vi "poly_run_vi_ref.vi"(8 "Error in":errorcluster caption="Error in (no error)", 9 "Auto dispose VI refnum?":bool=TRUE caption="Auto dispose VI refnum? (T)", 10 "Wait until VI done?":bool caption="Wait until VI done? (F)", 11 "VI refnum in":refnum<vi>) -> (0 "Error out":errorcluster, 1 "Was running?":bool, 2 "VI running?":bool, 3 "VI refnum out":refnum<vi>, 4 "Last execution state":T1(ring))   [LabVIEW 2015, in "_ref_tools_polys.lvlib"]
doc: "Runs the VI that <B>VI refnum in</B> refers to.\n\nThis function will wait until the VI is done if <B>Wait until VI done?</B> is True (default is False), and it will auto dispose the VI reference (hand it over to the running VI) if <B>Auto dispose VI refnum?</B> is True.\n\nThe VI must already be in memory (execution state \"Idle\" or \"Running\") for this function to take any action.\n\nThe <B>VI running?</B> output will only be True if the VI's <B>Last execution state</B> is \"Run top level\". Note that if this function fails to run the VI, <B>VI refnum in</B> will not be auto-disposed, in which case you retain the responsibility of closing that reference yourself.\n\nThis VI is reentrant, and it doesn't run if there is an error on <B>Error in</B>.\n\nSteen Schmidt\nGPower\n30/12 2012"
uses:
  _ref_tools_polys.lvlib
  poly_is_running_state.vi
panel:
  # "Based on Steen Schmidt's GPower"
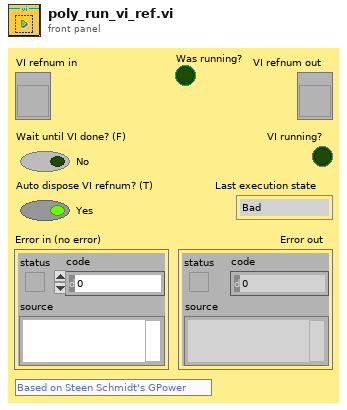
[diagram p1: front panel]
types:
  T1 = enum32{"Bad", "Idle", "Run top level", "Running"}
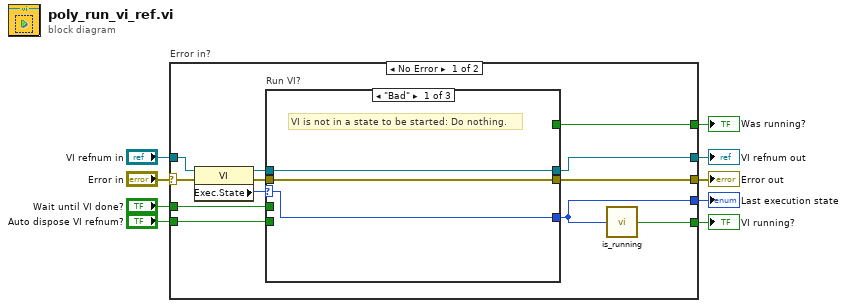
[diagram p0: block diagram]
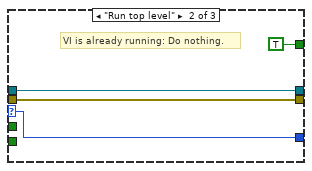
[diagram p2: hidden frame]
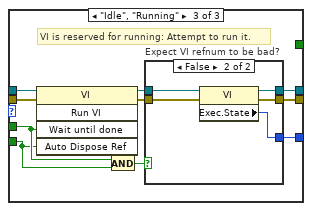
[diagram p3: hidden frame]
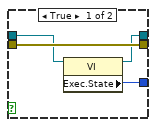
[diagram p4: hidden frame]
diagram:
  n1 = case "Error in?" shown="No Error" "Error in" {
    selector: "Error in" -> [w19 w48]
    tunnel: [w21 w48] -> w8
    tunnel: "VI refnum in" -> [w17 w49]
    tunnel: [w20 w49] -> w6
    tunnel: [w11 _] -> w5
    tunnel: [w10 _] -> w4
    tunnel: "Auto dispose VI refnum?" -> [w14 _]
    tunnel: "Wait until VI done?" -> [w13 _]
    tunnel: [w12 _] -> w1
    frame No Error {
      n2 = property class="VI"(reference=w17, error in=w19) -> (reference out=w16:refnum<vi>, error out=w18:errorcluster, "Exec.State"=w15:T1)
      n3 = case "Run VI?" shown="\"Bad\"" w15 {
        selector: w15 -> [w22 w26 _]
        tunnel: [w24 w28 w35] -> w21
        tunnel: w18 -> [w24 w28 w38]
        tunnel: w16 -> [w23 w27 w37]
        tunnel: [w23 w27 w33] -> w20
        tunnel: [w22 w26 w32] -> w11
        tunnel: w14 -> [_ _ w30]
        tunnel: w13 -> [_ _ w31]
        tunnel: [_ TRUE _] -> w12
        frame "Bad" {
          # "VI is not in a state to be started: Do nothing."
        }
        frame "Run top level" {
          # "VI is already running: Do nothing."
        }
        frame "Idle", "Running" {
          # "VI is reserved for running: Attempt to run it."
          n4 = invoke on="Run VI" class="VI" method="Run VI"(reference=w37, error in=w38, "Wait until done"=w31, "Auto Dispose Ref"=w30) -> (reference out=w34:refnum<vi>, error out=w36:errorcluster)  [unwired: 1 in, 3 out]
          n5 = And(x=w31, y=w30) -> (x .and. y?=w29:bool)
          n6 = case "Expect VI refnum to be bad?" shown="False" w29 {
            tunnel: w36 -> [w42 w47]
            tunnel: [w42 w46] -> w35
            tunnel: w34 -> [w41 w45]
            tunnel: [w39 w44] -> w33
            tunnel: [w40 w43] -> w32
            frame True {
              n7 = property class="VI"(reference=w41) -> (reference out=w39:refnum<vi>, "Exec.State"=w40:T1)  [unwired: 1 in, 1 out]
            }
            frame False {
              n8 = property class="VI"(reference=w45, error in=w47) -> (reference out=w44:refnum<vi>, error out=w46:errorcluster, "Exec.State"=w43:T1)
            }
          }
        }
      }
      n9 = call-poly "is_running.vi"("execution state"=w11) -> ("running top level?"=w10:bool)  [unwired: 4 in]
    }
    frame Error {
    }
  }
  "Error out" <- w8
  "VI refnum out" <- w6
  "Last execution state" <- w5
  "VI running?" <- w4
  "Was running?" <- w1
